vi "_Read VAC Gauge.vi"() -> (0 "DAC":u8)   [LabVIEW 2012]
uses:
  <vilib>/eio/EIONode/EIONode.xnode
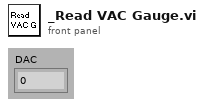
[diagram p1: front panel]
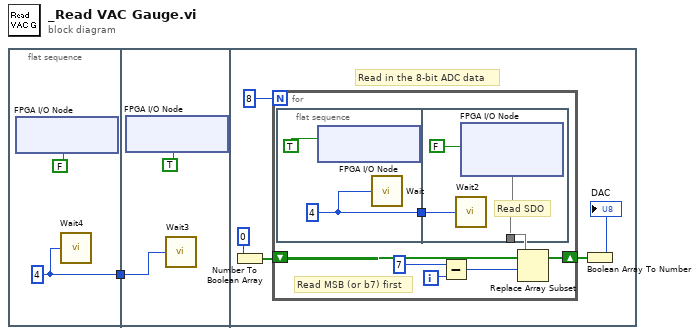
[diagram p0: block diagram]
diagram:
  n1 = flat-sequence {
    tunnel: [w2] -> w1
    tunnel: w1 -> [w4]
    frame #0 {
      w2 = u8 4 ("Count(uSec)")
      n2 = xnode "FPGA I/O Node"("Port6/DIO4"=FALSE ("Clock")) -> ()  [unwired: 1 in, 1 out]
      n3 = call "Wait4"("Count(Ticks)"=w2) -> ()  [unwired: 1 out]
    }
    frame #1 {
      n4 = xnode "FPGA I/O Node"("Port6/DIO4"=TRUE ("Clock")) -> ()  [unwired: 1 in, 1 out]
      n5 = call "Wait3"("Count(uSec)"=w4) -> ()  [unwired: 1 out]
    }
    frame #2 {
      # "Read in the 8-bit ADC data"
      n6 = Number To Boolean Array(number=u8 0) -> (Boolean array=w8:bool[])
      n7 = for {
        N: 8 -> [_]
        shift-right: [w16] -> w7
        shift-left: w8 -> [w17]
        i -> [w15]
        # "Read MSB (or b7) first"
        n8 = flat-sequence {
          tunnel: [w18] -> w11
          tunnel: [w22] -> w12
          tunnel: w11 -> [w20]
          frame #0 {
            w18 = u8 4 ("Count(Ticks)")
            n9 = xnode "FPGA I/O Node"("Port6/DIO5"=TRUE ("Clock")) -> ()  [unwired: 1 in, 1 out]
            n10 = call "Wait"("Count(Ticks)"=w18) -> ()  [unwired: 1 out]
          }
          frame #1 {
            # "Read SDO"
            n11 = call "Wait2"("Count(Ticks)"=w20) -> ()  [unwired: 1 out]
            n12 = xnode "FPGA I/O Node"("Port6/DIO5"=FALSE ("Clock")) -> ("Port6/DIO6"=w22)  [unwired: 2 in, 2 out]
          }
        }
        n13 = Subtract(x=7, y=w15) -> (x-y=w13:i32)
        n14 = Replace Array Subset(array=w17, new element=w12, index=w13) -> (w16:bool[])
      }
      n15 = Boolean Array To Number(Boolean array=w7) -> (number=→"DAC":u8)
    }
  }
